vi "ImageCopy.vi"() -> (0 "ErrOut":errorcluster)   [LabVIEW 2014]
doc: "Use this template to build a VI to use as a subVI."
panel:
  out "Image":T1(plugin-control)
  out "Custom Data Out":string
  in  "ErrIn":errorcluster
  # "Input Parameters"
  # "Output Parameters"
  # "VI Description:\nThis VI is .."
  # ":: MVI Framework V1.0 ::\nAuthor:Gaoke Yang\nEmail: gaoke.yang@yahoo.com\nWeb: www.mvicontrol.com\nCopyright (C) 2013, MVI Technologies All Rights Reserved"
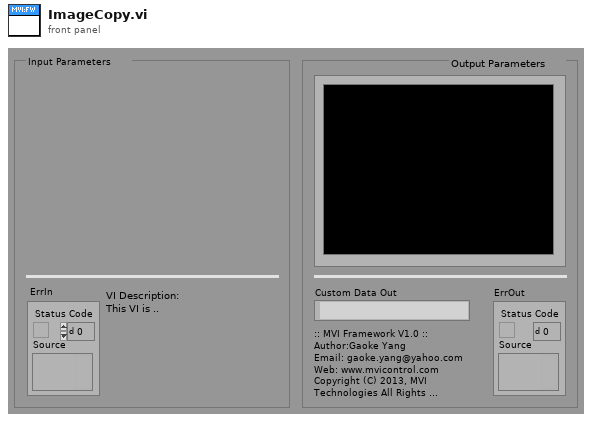
[diagram p1: front panel]
types:
  T1 = typedef "IMAQ Image.ctl" = refnum<image>
  T2 = typedef "Image Type" = u32
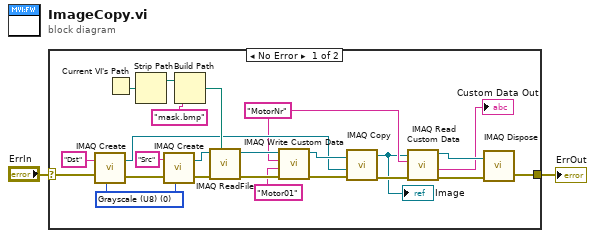
[diagram p0: block diagram]
diagram:
  n1 = case shown="No Error" "ErrIn" {
    selector: "ErrIn" -> [w17 w27]
    tunnel: [w25 w27] -> w2
    frame No Error {
      w4 = "MotorNr" ("Key")
      w13 = T2 0 items=["Grayscale (U8)", "Grayscale (I16)", "Grayscale (SGL)", "Complex (CSG)", "RGB (U32)", "HSL (U32)", "RGB (U64)", "Grayscale (U16)"] ("Image Type")
      n2 = call "IMAQ Create"("Image Name"="Dst", "Image Type"=w13, "error in (no error)"=w17) -> ("New Image"=w6:T1, "error out"=w12:errorcluster)  [unwired: 2 in]
      n3 = Current VI's Path() -> (path=w23:path)
      n4 = Strip Path(path=w23) -> (stripped path=w22:path)  [unwired: 1 out]
      n5 = call "IMAQ Create"("Image Name"="Src", "Image Type"=w13, "error in (no error)"=w12) -> ("New Image"=w9:T1, "error out"=w10:errorcluster)  [unwired: 2 in]
      n6 = Build Path(base path=w22, name or relative path="mask.bmp") -> (appended path=w21:path)
      n7 = call "IMAQ ReadFile"("File Path"=w21, "error in (no error)"=w10, "Image"=w9) -> ("error out"=w19:errorcluster, "Image Out"=w20:T1)  [unwired: 4 in, 3 out]
      n8 = call "IMAQ Write Custom Data"("error in (no error)"=w19, "Custom Data In"="Motor01", "Key"=w4, "Image"=w20) -> ("error out"=w8:errorcluster, "Image Out"=w7:T1)  [unwired: 6 in]
      n9 = call "IMAQ Copy"("error in (no error)"=w8, "Image Dst"=w6, "Image Src"=w7) -> ("error out"=w5:errorcluster, "Image Dst Out"=w3:T1)  [unwired: 3 in]
      "Image" <- w3
      n10 = call "IMAQ Read Custom Data"("error in (no error)"=w5, "Key"=w4, "Image"=w3) -> ("error out"=w16:errorcluster, "Custom Data Out"=→"Custom Data Out":string, "Image (duplicate)"=w15:T1)  [unwired: 6 in]
      n11 = call "IMAQ Dispose"("Image"=w15, "error in (no error)"=w16) -> ("error out"=w25:errorcluster)  [unwired: 4 in]
    }
    frame Error {
    }
  }
  "ErrOut" <- w2
